vi "Read DAQ FIFO.vi"(8 "error in (no error)":errorcluster, 9 "Timeout (ms)":i32, 10 "Data In":T1[](array[typedef]), 11 "CIFFIFO in":refnum<class "CIF_CIPC_Fifo_DAQ.lvclass">) -> (0 "error out":errorcluster, 1 "timed out?":bool, 2 "Data Out":T1[](array[typedef]), 3 "CIFFIFO out":refnum<class "CIF_CIPC_Fifo_DAQ.lvclass">, 4 "Header":T2)   [LabVIEW 2021, in "CIF_CIPC_Fifo_DAQ.lvclass"]
uses:
  CIF_CIPC_Fifo_DAQ.lvclass
  ChannelCommon/typedef/FIFO Header.ctl
  D:/dev/Packages/CIF_Channels_Core/src/CIFChannels/CIFChannels.lvclass
  D:/dev/Packages/CIF_Channels_Core/src/CIPC_Channels/CIF_CIPC_Chan/CIF_CIPC_Chn.lvclass
  ChannelCommon/typedef/Datatype Waveform.ctl
  CIFChannels/CIFChannels.lvclass/CIFChannels.ctl
  CIF_CIPC_Chan/CIF_CIPC_Chn.lvclass/CIF_CIPC_Chn.ctl
  CIF_CIPC_Fifo_DAQ.lvclass/CIF_CIPC_Fifo_DAQ.ctl
  <vilib>/CIF Foundation/CIF Utilities/Statistics/I64/Stats_I64_CIF_U.lvclass/Stats_I64_CIF_U.ctl
  CIFChannels/Accessors/Read FIFO Header.vi
  ChannelCommon/Utilities/Unflatten Header.vi
  CIFChannels/Accessors/Write FIFO Header.vi
  ChannelCommon/Utilities/Remove Header Bytes.vi
  SubVIs/Read One DAQ Waveform.vi
  SubVIs/Read Wrapper for BP U8.vi
  CIFChannels/Utilities/Update Channel Benchmark.vi
  SubVIs/Core Read DAQ FIFO.vi/e703c505-0034-46a9-8989-21c0de27793f.vi
  SubVIs/Core Read DAQ FIFO.vi/768488f4-e6df-4560-a449-a64b33b49031.vi
  CIFChannels/Accessors/Read Channel State.vi
  CIFChannels/Accessors/Read Direction.vi
  <vilib>/CIF Foundation/CIF Utilities/DataTypes/Flatten Unflatten/Unflatten U64.vi
  <vilib>/CIF Foundation/CIF Utilities/DataTypes/Flatten Unflatten/Unflatten I64.vi
  ChannelCommon/Utilities/Add Error.vi
  SubVIs/Read Wrapper for BP Meta.vi
  SubVIs/Read Wrapper for BP Measurements.vi
  CIF_CIPC_Chan/Accessors/Read CIPC Channel.vi
  SubVIs/Read Wrapper for BP U8.vi/b5615cf0-cd7f-4476-b9a9-d6ef7628cc3b.vi
  CIF_CIPC_Chan/Accessors/Read Buffer Configuration.vi
  SubVIs/Read Wrapper for BP U8.vi/6248fc70-cc83-4025-b778-a3221b95feac.vi
  CIFChannels/Accessors/Read FIFO Backpressure.vi
  <vilib>/CIF Foundation/CIF Utilities/Statistics/I64/X1 minus X0.vi
  <vilib>/CIF Foundation/CIF Utilities/Time/System Time/Get System Time.vi
  SubVIs/Read Wrapper for BP Meta.vi/b5615cf0-cd7f-4476-b9a9-d6ef7628cc3b.vi
  SubVIs/Read Wrapper for BP Meta.vi/6248fc70-cc83-4025-b778-a3221b95feac.vi
  SubVIs/Read Wrapper for BP Measurements.vi/b5615cf0-cd7f-4476-b9a9-d6ef7628cc3b.vi
  SubVIs/Read Wrapper for BP Measurements.vi/6248fc70-cc83-4025-b778-a3221b95feac.vi
  <vilib>/CIF Foundation/CIF CIPC/SubVIs/Wait For N Elements Available.vi
  <vilib>/CIF Foundation/CIF CIPC/SubVIs/Get Element Read Position.vi
  <vilib>/CIF Foundation/CIF CIPC/SubVIs/Check Error.vi
  <vilib>/CIF Foundation/CIF CIPC/SubVIs/Get dll Path.vi
  <vilib>/CIF Foundation/CIF CIPC/SubVIs/Set Element Read Position.vi
  SubVIs/Read Wrapper for BP U8.vi/6248fc70-cc83-4025-b778-a3221b95feac.vi/331f6ecb-7ec4-4931-b93d-4fbd8d66a851.vi
  SubVIs/Read Wrapper for BP U8.vi/6248fc70-cc83-4025-b778-a3221b95feac.vi/5ce0d4cf-f921-42ba-b14c-c90f7f7611e4.vi
  <vilib>/CIF Foundation/CIF Utilities/Statistics/I64/X1 minus X0.vi/dfabcf33-0dbc-4041-80a5-3dc0c86d2989.vi
  <vilib>/CIF Foundation/CIF Utilities/Time/System Time/LabVIEW Time to TAI Time.vi
  SubVIs/Read Wrapper for BP Meta.vi/6248fc70-cc83-4025-b778-a3221b95feac.vi/331f6ecb-7ec4-4931-b93d-4fbd8d66a851.vi
  SubVIs/Read Wrapper for BP Meta.vi/6248fc70-cc83-4025-b778-a3221b95feac.vi/5ce0d4cf-f921-42ba-b14c-c90f7f7611e4.vi
  SubVIs/Read Wrapper for BP Measurements.vi/6248fc70-cc83-4025-b778-a3221b95feac.vi/331f6ecb-7ec4-4931-b93d-4fbd8d66a851.vi
  SubVIs/Read Wrapper for BP Measurements.vi/6248fc70-cc83-4025-b778-a3221b95feac.vi/5ce0d4cf-f921-42ba-b14c-c90f7f7611e4.vi
  <vilib>/CIF Foundation/CIF CIPC/SubVIs/Notify Of New Write.vi
  <vilib>/CIF Foundation/CIF CIPC/SubVIs/Get Element Write Position.vi
  <vilib>/CIF Foundation/CIF Utilities/Statistics/I64/X1 minus X0.vi/dfabcf33-0dbc-4041-80a5-3dc0c86d2989.vi/9eb60a9a-770f-4d2d-8b3f-8465c267ecc9.vi
  <vilib>/CIF Foundation/CIF CIPC/SubVIs/Check Error Core.vi
  <vilib>/CIF Foundation/CIF CIPC/SubVIs/Get Element Info Variant.vi
  ChannelCommon/Utilities/Add Error Core.vi
  ChannelCommon/ChannelCommon.lvlib
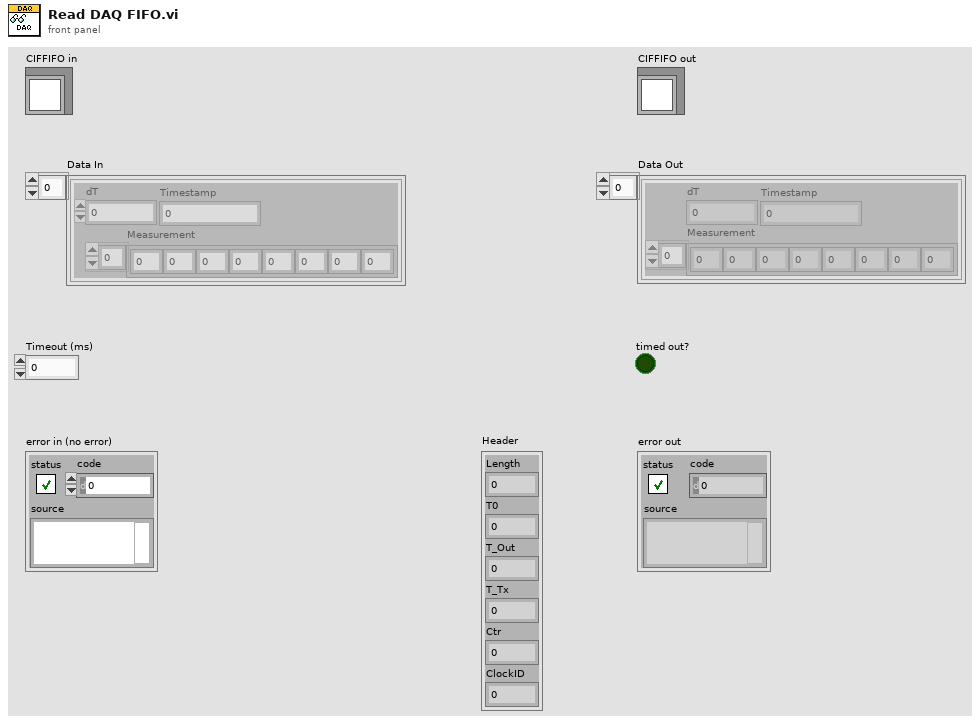
[diagram p1: front panel]
types:
  T1 = typedef "ChannelCommon.lvlib/Datatype Waveform.ctl" = cluster{"Measurement":dbl[], "dT":dbl, "Timestamp":i64}
  T2 = typedef "ChannelCommon.lvlib/FIFO Header.ctl" = cluster{"Length":u64, "T0":i64, "T_Out":i64, "T_Tx":i64, "Ctr":u64, "ClockID":u8}
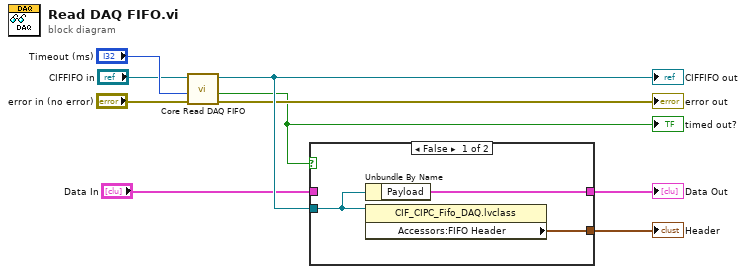
[diagram p0: block diagram]
diagram:
  n1 = call "Core Read DAQ FIFO.vi"("error in (no error)"="error in (no error)", "Timeout (ms)"="Timeout (ms)", "CIFFIFO in"="CIFFIFO in") -> ("error out"=→"error out":errorcluster, "timed out?"=w3:bool, "CIFFIFO out"=w5:refnum<class "CIF_CIPC_Fifo_DAQ.lvclass">)  [unwired: 6 in]
  "timed out?" <- w3
  "CIFFIFO out" <- w5
  n2 = case shown="False" w3 {
    tunnel: w5 -> [w12 _]
    tunnel: [w10 w13] -> w1
    tunnel: [w11 _] -> w7
    tunnel: "Data In" -> [_ w13]
    frame False {
      n3 = Unbundle By Name(w12) -> ("Payload"=w10:T1[])
      n4 = property class="CIF_CIPC_Fifo_DAQ.lvclass"(reference=w12) -> ("Accessors:FIFO Header"=w11:T2)  [unwired: 1 in, 2 out]
    }
    frame True {
    }
  }
  "Header" <- w7
  "Data Out" <- w1
